vi "ASIC_WRITE.vi"(0 "ftHandle_in":u32, 1 "Espera acceso USB":u32=10, 5 "Direccion Registro Asic":u8 format="%x", 7 "Byte Alto":u8 format="%x", 9 "Byte Bajo":u8 format="%x", 11 "error in":errorcluster) -> (4 "ftHandle_out":u32, 15 "error out":errorcluster)   [LabVIEW 2019]
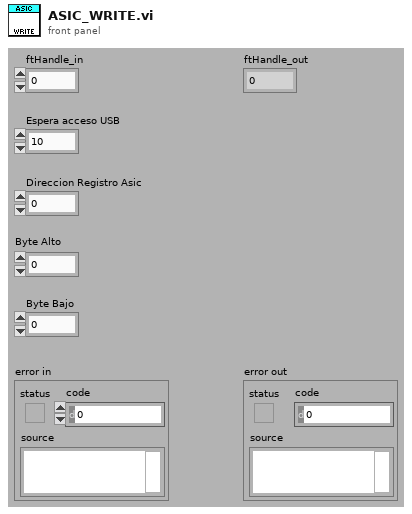
[diagram p1: front panel]
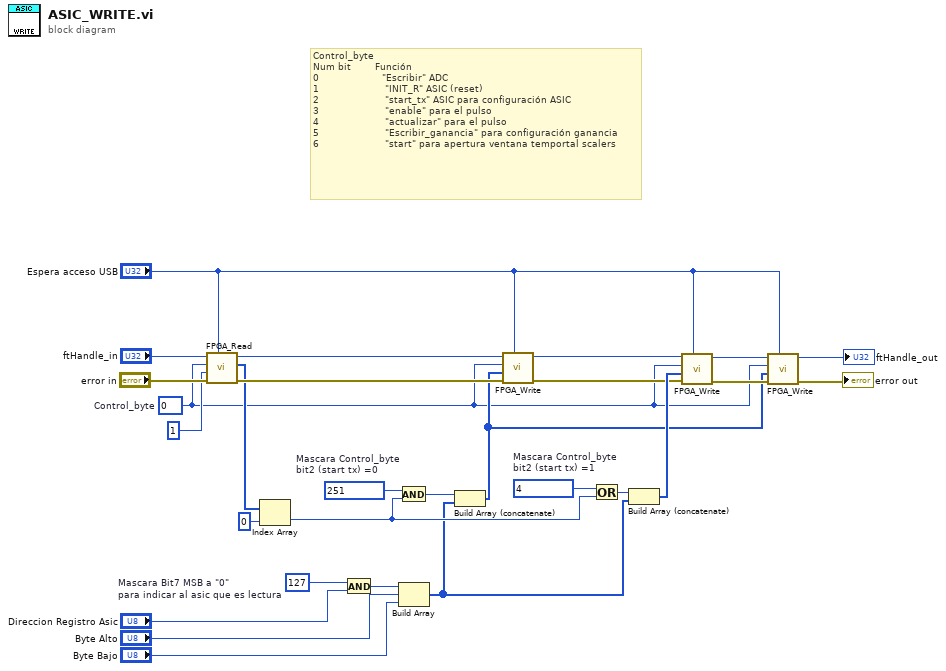
[diagram p0: block diagram]
diagram:
  w13 = u8 4  # Mascara Control_byte bit2 (start tx) =1
  w27 = u8 127  # Mascara Bit7 MSB a "0" para indicar al asic que es lectura
  w2 = u8 0  # Control_byte
  w20 = u8 251  # Mascara Control_byte bit2 (start tx) =0
  # "Control_byte\nNum bit        Función\n0                     \"Escribir\" ADC\n1                      \"INIT_R\" ASIC (reset)\n2                      \"start_tx\" ASIC para configuración ASIC\n3                      \"enable\" para el pulso\n4                      \"actualizar\" para el pulso\n5                      \"Escribir_ganancia\" para configuración ganancia\n6                      \"start\" para apertura ventana temportal scalers"
  n1 = call "FPGA_Read.vi"("Espera acceso USB"="Espera acceso USB", "error in"="error in", "Numero Bytes"=u8 1, "Dirección base"=w2, "ftHandle_in"="ftHandle_in") -> ("error out"=w24:errorcluster, "lpBuffer_out"=w22:u8[], "ftHandle_out"=w1:u32)  [unwired: 2 in, 2 out]
  n2 = Index Array(array=w22, index=0) -> (element=w14:u8)
  n3 = And(x=w27, y="Direccion Registro Asic") -> (x .and. y?=w18:u8)
  n4 = And(x=w20, y=w14) -> (x .and. y?=w15:u8)
  n5 = Build Array ("Escribimos en usb reg1, reg2, reg3 y reg4")(w18, "Byte Alto", "Byte Bajo") -> (w9:u8[])
  n6 = Build Array (concatenate) ("Escribimos en usb reg1, reg2, reg3 y reg4")(w15, w9) -> (w3:u8[])
  n7 = call "FPGA_Write.vi"("Espera acceso USB"="Espera acceso USB", "error in"=w24, "Bytes de escritura"=w3, "Dirección base"=w2, "ftHandle_in"=w1) -> ("error out"=w10:errorcluster, "ftHandle_out"=w19:u32)  [unwired: 1 in, 2 out]
  n8 = Or(x=w13, y=w14) -> (x .or. y?=w12:u8)
  n9 = Build Array (concatenate) ("Escribimos en usb reg1, reg2, reg3 y reg4")(w12, w9) -> (w11:u8[])
  n10 = call "FPGA_Write.vi"("Espera acceso USB"="Espera acceso USB", "error in"=w10, "Bytes de escritura"=w11, "Dirección base"=w2, "ftHandle_in"=w19) -> ("error out"=w7:errorcluster, "ftHandle_out"=w8:u32)  [unwired: 1 in, 2 out]
  n11 = call "FPGA_Write.vi"("Espera acceso USB"="Espera acceso USB", "error in"=w7, "Bytes de escritura"=w3, "Dirección base"=w2, "ftHandle_in"=w8) -> ("error out"=→"error out":errorcluster, "ftHandle_out"=→"ftHandle_out":u32)  [unwired: 1 in, 2 out]
